vi "GD TimeStamp.vi"(11 "Zeitformatierungs-String (%c)":string="%Y-%m-%d %H:%M:%S ") -> (2 "date/time string":string, 3 "current time":timestamp)   [LabVIEW 2020, in "Linearisierung v2.lvlib" / "Gasteiler.lvlib"]
uses:
  Gasteiler.lvlib
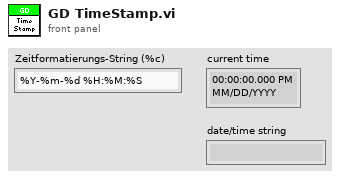
[diagram p1: front panel]
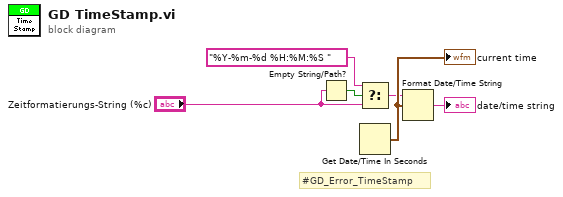
[diagram p0: block diagram]
diagram:
  # "#GD_Error_TimeStamp"
  n1 = Empty String/Path?(string/path="Zeitformatierungs-String (%c)") -> (empty?=w4:bool)
  n2 = Select(t="%Y-%m-%d %H:%M:%S " ("Zeitformatierungs-String (%c)"), s=w4, f="Zeitformatierungs-String (%c)") -> (s? t:f=w2:string)
  n3 = Get Date/Time In Seconds() -> (seconds since 1Jan1904=w6:timestamp)
  "current time" <- w6
  n4 = Format Date/Time String(time format string (%c)=w2, seconds (now)=w6) -> (date/time string=→"date/time string":string)  [unwired: 1 in]
